vi "Search Sysdef for Targets.vi"(8 "error in (no error)":errorcluster, 11 "NIVS.System Definition Root":refnum<k24>) -> (0 "error out":errorcluster, 1 "Target Names":string[](array[string]), 3 "NIVS.System Defintion Root Out":refnum<k24>, 7 "Target Nodes":refnum<k24>[](array[refnum]))   [LabVIEW 2015, in "J1939 Addon Shared.lvlib"]
uses:
  J1939 Addon Shared.lvlib
  NationalInstruments.VeriStand.SystemStorage
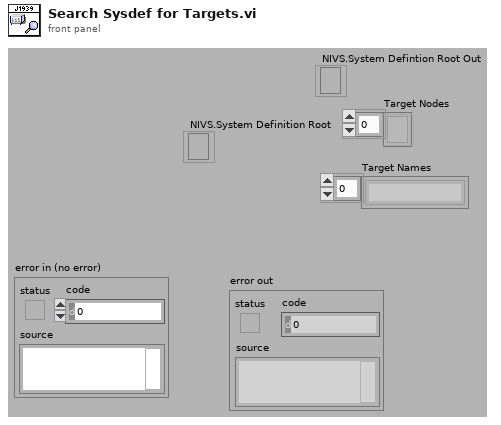
[diagram p1: front panel]
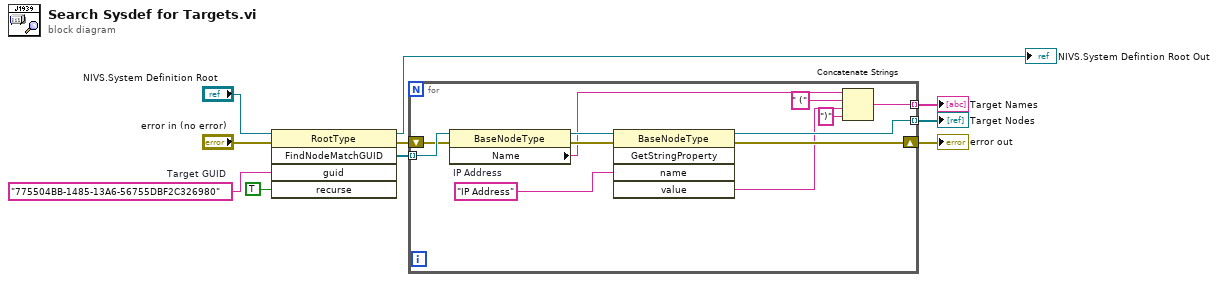
[diagram p0: block diagram]
diagram:
  w4 = "775504BB-1485-13A6-56755DBF2C326980"  # Target GUID
  n1 = invoke class="RootType" method="FindNodeMatchGUID"(reference="NIVS.System Definition Root", error in="error in (no error)", "guid"=w4, "recurse"=TRUE) -> (reference out=→"NIVS.System Defintion Root Out":refnum<k24>, error out=w2:errorcluster, "FindNodeMatchGUID"=w3:refnum<k24>[])  [unwired: 1 in, 2 out]
  n2 = for {
    tunnel: w3 -> [w22] mode=indexing
    shift-right: [w18] -> w5
    shift-left: w2 -> [w21]
    tunnel: [w17] -> w7 mode=indexing
    tunnel: [w11] -> w6 mode=indexing
    w16 = "IP Address"  # IP Address
    n3 = property class="BaseNodeType"(reference=w22, error in=w21) -> (reference out=w20:refnum<k24>, error out=w19:errorcluster, "Name"=w12:string)
    n4 = invoke class="BaseNodeType" method="GetStringProperty"(reference=w20, error in=w19, "name"=w16) -> (reference out=w17:refnum<k24>, error out=w18:errorcluster, "value"=w14:string)  [unwired: 2 in, 2 out]
    n5 = Concatenate Strings(w12, " (" ("string"), w14, ")" ("string")) -> (w11:string)
  }
  "error out" <- w5
  "Target Nodes" <- w7
  "Target Names" <- w6
